vi "DSB(SubVI).vi"(5 "mod index":dbl(slide)=1.0 scale=0.0..1.0, 6 "modulation frequency":dbl(knob)=10.0 scale=0.0..1000.0, 7 "sampling info":cluster{"Fs":dbl, "#s":dbl}, 8 "carrier frequency":dbl(knob)=10.0 scale=0.0..500000.0, 9 "carrier amplitude":dbl(slide) scale=0.0..10.0) -> (0 "baseband signal (frequency-domain)":cluster{"f0":dbl, "df":dbl, "magnitude":dbl[]}(graph), 1 "power ratio":dbl, 2 "modulated signal (frequency-domain)":cluster{"f0":dbl, "df":dbl, "magnitude":dbl[]}(graph), 3 "modulated signal (time-domain)":waveform(dbl)(graph), 4 "baseband signal (time-domain)":waveform(dbl)(graph))   [LabVIEW 2010]
uses:
  <vilib>/measure/maspectr.llb/FFT Spectrum (Mag-Phase) for 1 Chan.vi
  <vilib>/measure/NI_MABase.lvlib
  <vilib>/measure/NI_MAPro.lvlib
  <vilib>/ptbypt/NI_PtbyPt.lvlib
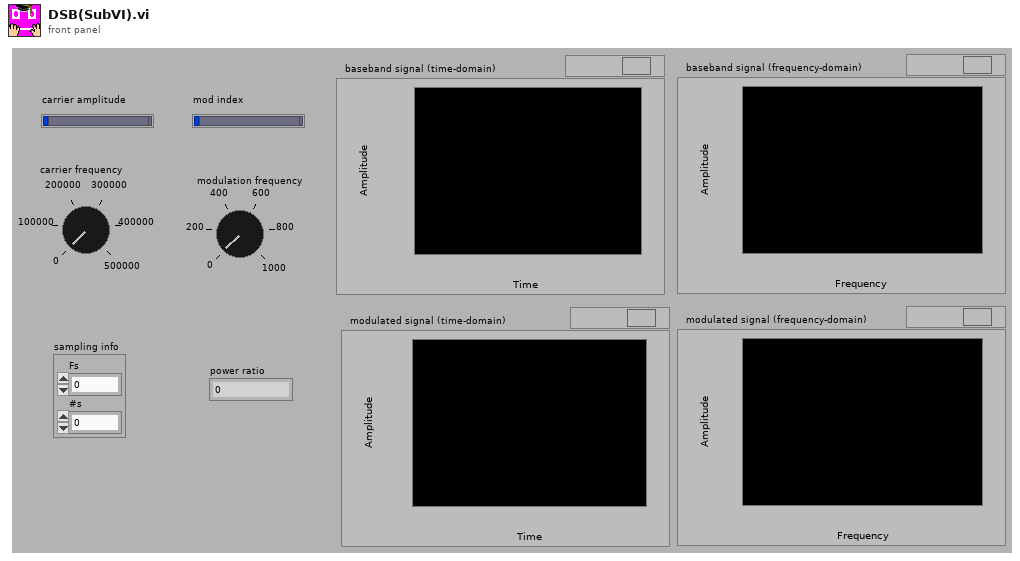
[diagram p1: front panel]
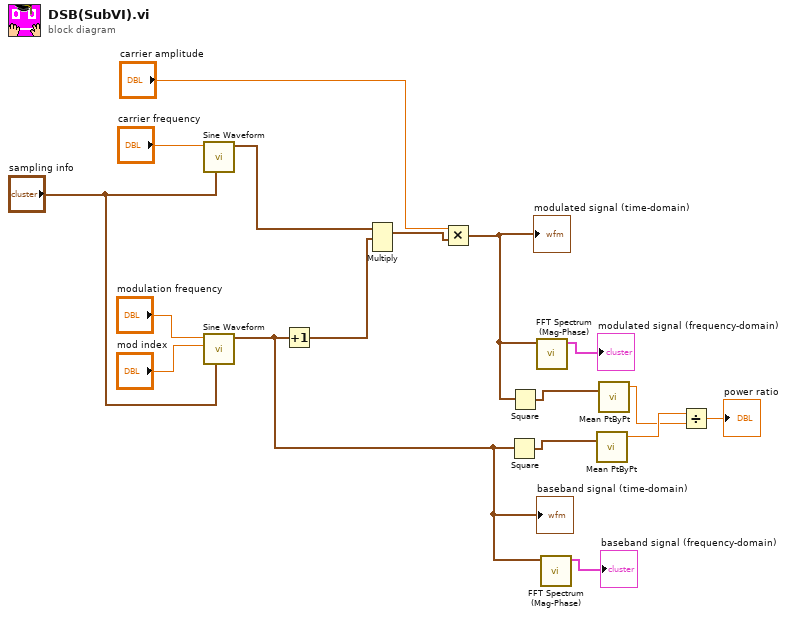
[diagram p0: block diagram]
diagram:
  n1 = call <vilib>:"Sine Waveform.vi"("sampling info"="sampling info", "frequency"="carrier frequency") -> ("signal out"=w11:waveform(dbl))  [unwired: 8 in, 1 out]
  n2 = call <vilib>:"Sine Waveform.vi"("sampling info"="sampling info", "amplitude"="mod index", "frequency"="modulation frequency") -> ("signal out"=w1:waveform(dbl))  [unwired: 7 in, 1 out]
  "baseband signal (time-domain)" <- w1
  n3 = Increment(x=w1) -> (x+1=w10:waveform(dbl))
  n4 = Multiply(1:w10, 2:w11) -> (0:w16:waveform(dbl))  [unwired: 1 in, 1 out]
  n5 = Multiply(x="carrier amplitude", y=w16) -> (x*y=w15:waveform(dbl))
  "modulated signal (time-domain)" <- w15
  n6 = Square(x=w1) -> (x^2=w8:waveform(dbl))
  n7 = Square(x=w15) -> (x^2=w7:waveform(dbl))
  n8 = call-poly <vilib>:"FFT Spectrum (Mag-Phase).vi"("time signal"=w15) -> ("magnitude"=→"modulated signal (frequency-domain)":cluster{"f0":dbl, "df":dbl, "magnitude":dbl[]})  [unwired: 6 in, 4 out]
  n9 = call-poly <vilib>:"FFT Spectrum (Mag-Phase).vi"("time signal"=w1) -> ("magnitude"=→"baseband signal (frequency-domain)":cluster{"f0":dbl, "df":dbl, "magnitude":dbl[]})  [unwired: 6 in, 4 out]
  n10 = call <vilib>:"Mean PtByPt.vi"("x"=w8) -> ("mean"=w5:dbl)  [unwired: 3 in, 1 out]
  n11 = call <vilib>:"Mean PtByPt.vi"("x"=w7) -> ("mean"=w4:dbl)  [unwired: 3 in, 1 out]
  n12 = Divide(x=w5, y=w4) -> (x/y=→"power ratio":dbl)
